vi "The ChapR.vi"(8 "Digtl In":u8, 9 "Position":u8=49, 10 "Alliance":u8=66, 11 "TeamNo":u16) -> ()   [LabVIEW 2013]
uses:
  ChapR Packet.ctl
  <vilib>/Instr/_visa.llb/VISA Configure Serial Port (Instr).vi
panel:
  out "error out 3":errorcluster
  in  "connection ID":refnum<k16>
  out "error out 2":errorcluster
  out "# elements 2":u32
  out "# elements":u32
  out "error out":errorcluster
  out "value 2":T1
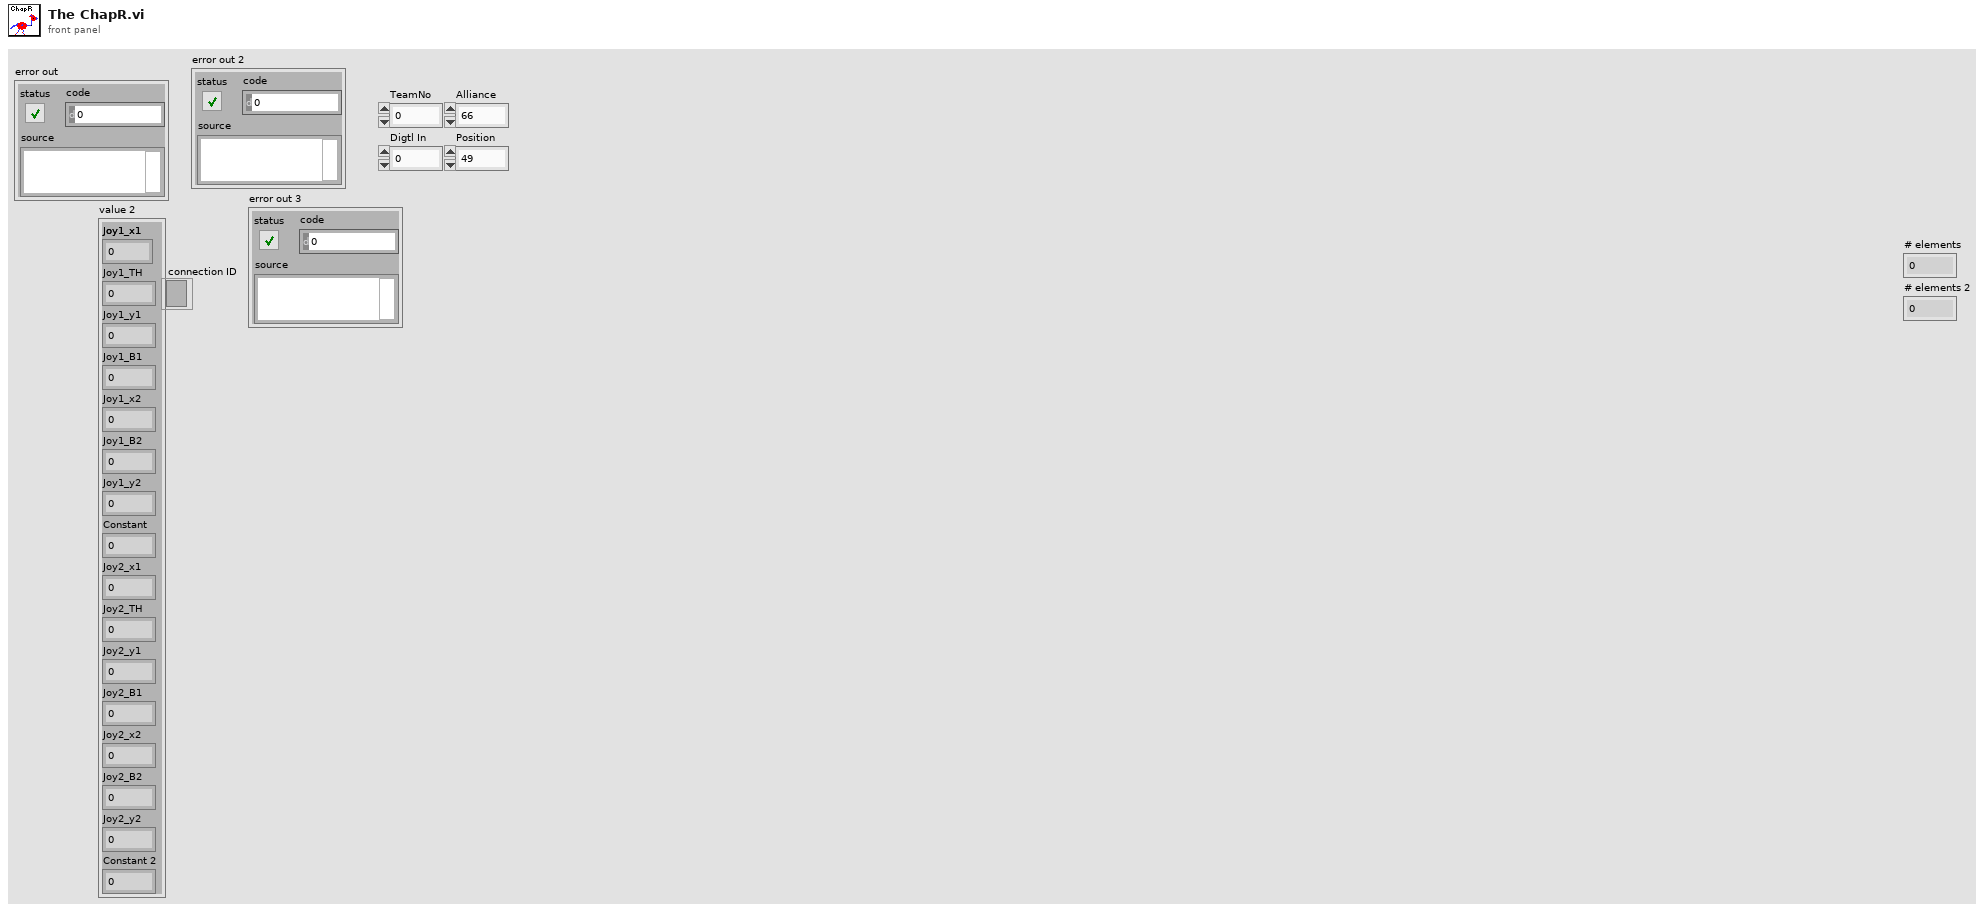
[diagram p1: front panel]
types:
  T1 = typedef "ChapR Packet.ctl" = cluster{"Joy1_x1":i8, "Joy1_TH":u8, "Joy1_y1":i8, "Joy1_B1":u8, "Joy1_x2":i8, "Joy1_B2":u8, "Joy1_y2":i8, "Constant":u8, "Joy2_x1":i8, "Joy2_TH":u8, "Joy2_y1":i8, "Joy2_B1":u8, "Joy2_x2":i8, "Joy2_B2":u8, "Joy2_y2":i8, "Constant 2":u8}
  T2 = cluster{"read mode":enum16{"polling", "blocking"}, "write mode":enum16{"polling", "blocking"}}
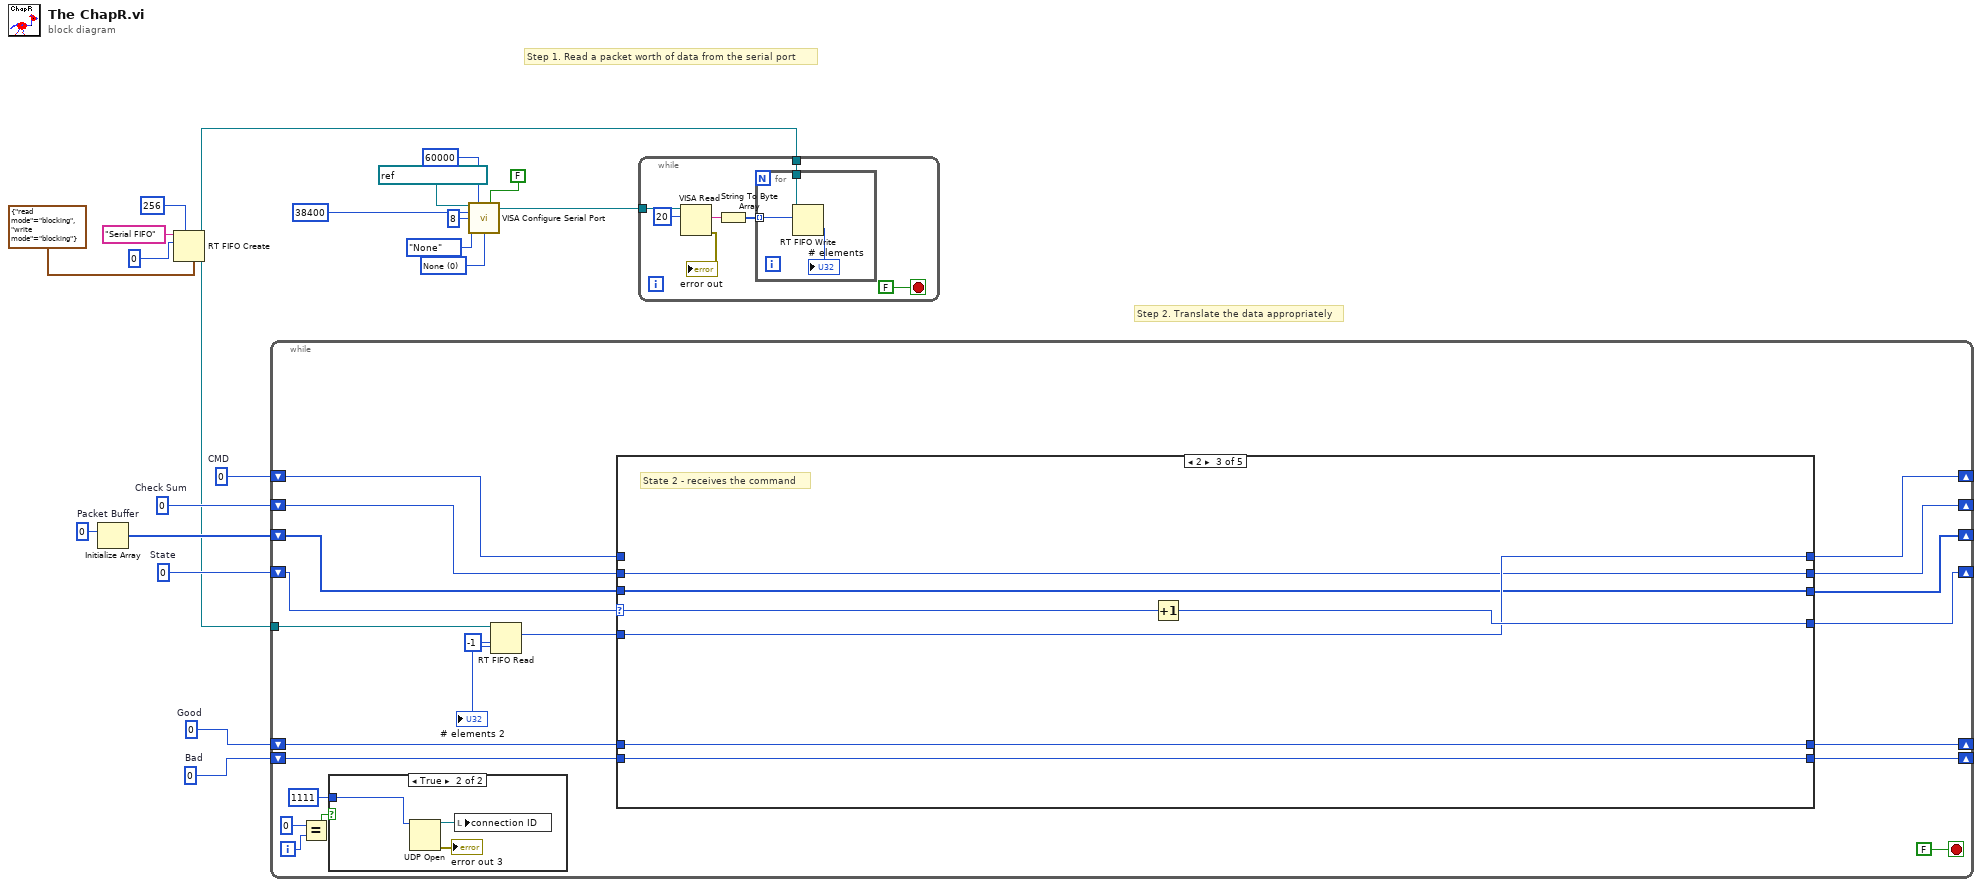
[diagram p0: block diagram]
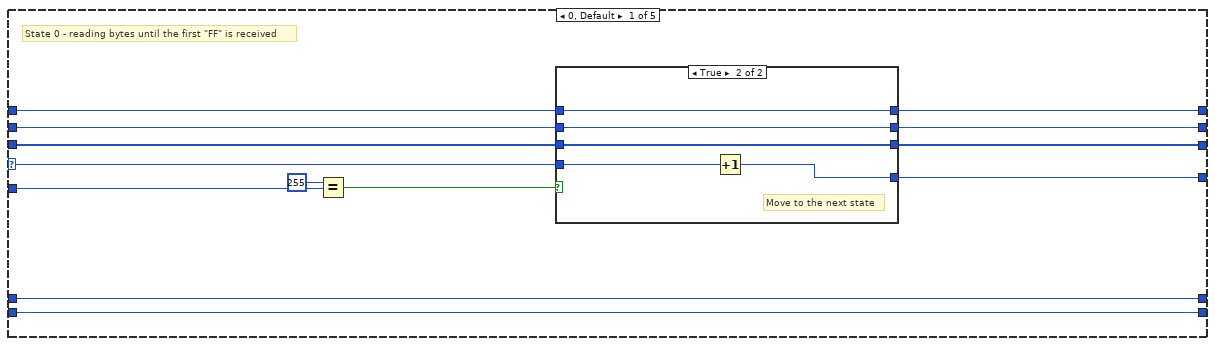
[diagram p3: hidden frame]
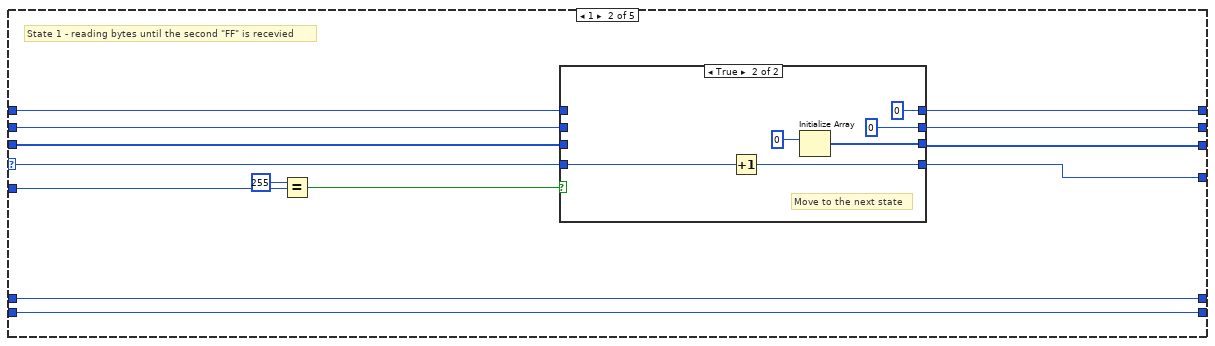
[diagram p5: hidden frame]
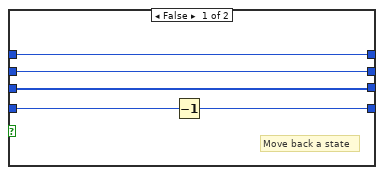
[diagram p6: hidden frame]
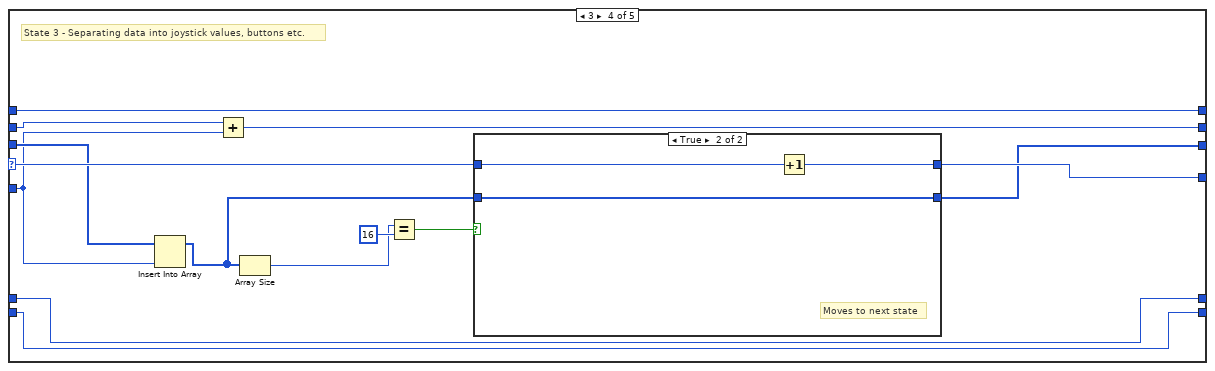
[diagram p7: hidden frame]
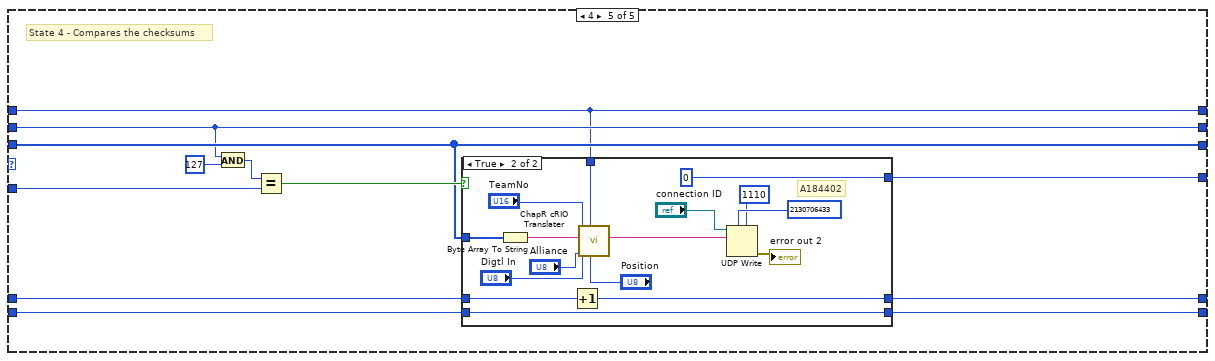
[diagram p9: hidden frame]
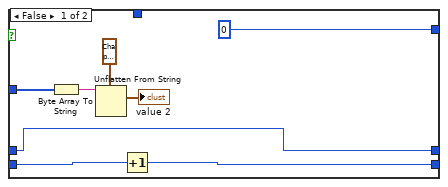
[diagram p10: hidden frame]
diagram:
  w5 = 0  # Bad
  w6 = 0  # Good
  w19 = u16 0 items=["None", "XON/XOFF", "RTS/CTS", "XON/XOFF & RTS/CTS", "DTR/DSR", "XON/XOFF & DTR/DSR"] ("flow control (0:none)")
  w3 = u8 0  # CMD
  w4 = u8 0  # Check Sum
  w20 = 0  # State
  # "Step 2. Translate the data appropriately"
  # "Step 1. Read a packet worth of data from the serial port"
  n1 = Initialize Array "Packet Buffer"(u8 0 ("element")) -> (w8:u8[])  [unwired: 1 in]
  n2 = RT FIFO Create(0:"Serial FIFO" ("name (unnamed)"), 1:u8 0 ("datapoints in waveform (1)"), 4:u32 256 ("size (10)"), 7:T2 {"read mode"=enum."blocking", "write mode"=enum."blocking"} ("r/w modes (polling,polling)")) -> (8:w1:refnum<k33>)  [unwired: 4 in, 2 out]
  n3 = while {
    shift-right: [w39] -> _
    shift-left: w20 -> [w40]
    shift-right: [w29] -> _
    shift-left: w4 -> [w30]
    tunnel: w1 -> [w37]
    shift-right: [w35] -> _
    shift-left: w8 -> [w36]
    shift-right: [w31] -> _
    shift-left: w6 -> [w34]
    shift-right: [w32] -> _
    shift-left: w5 -> [w33]
    shift-right: [w27] -> _
    shift-left: w3 -> [w28]
    i -> [w23]
    stop <- FALSE stop-if-true
    n4 = Equal?(x=0, y=w23) -> (x = y?=w24:bool)
    n5 = case shown="True" w24 {
      tunnel: u16 1111 ("port") -> [_ w43]
      frame False {
      }
      frame True {
        n6 = UDP Open(11:w43) -> (port=w44:refnum<k16>, 0:→"error out 3":errorcluster)  [unwired: 4 in, 1 out]
        n7 = local write "connection ID"(w44) -> ()
      }
    }
    n8 = RT FIFO Read(0:w37, 2:-1 ("timeout in ms (0)")) -> (7:→"# elements 2":u32, 9:w38:u8)  [unwired: 2 in, 3 out]
    n9 = case shown="2" w40 {
      selector: w40 -> [w56 w79 w97 w110 _]
      tunnel: [w55 w78 w96 w111 w127] -> w39
      tunnel: [w47 w69 w91 w108 w118] -> w29
      tunnel: [w45 w67 w95 w98 w117] -> w27
      tunnel: w38 -> [w53 w75 w95 w106 w124]
      tunnel: w36 -> [w52 w73 w94 w107 w123]
      tunnel: [w51 w74 w94 w102 w123] -> w35
      tunnel: w34 -> [w50 w72 w93 w101 w120]
      tunnel: w33 -> [w49 w71 w92 w100 w122]
      tunnel: [w49 w71 w92 w100 w121] -> w32
      tunnel: [w50 w72 w93 w101 w119] -> w31
      tunnel: w30 -> [w48 w70 w91 w99 w118]
      tunnel: w28 -> [w46 w68 _ w98 w117]
      frame 0, Default {
        # "State 0 - reading bytes until the first \"FF\" is received"
        n10 = Equal?(x=u8 255, y=w53) -> (x = y?=w57:bool)
        n11 = case shown="True" w57 {
          tunnel: w56 -> [w61 w66]
          tunnel: [w61 w65] -> w55
          tunnel: w52 -> [w60 w64]
          tunnel: [w60 w64] -> w51
          tunnel: [w59 w63] -> w47
          tunnel: w48 -> [w59 w63]
          tunnel: [w58 w62] -> w45
          tunnel: w46 -> [w58 w62]
          frame False {
            # "Do nothing"
          }
          frame True {
            # "Move to the next state"
            n12 = Increment(x=w66) -> (x+1=w65:i32)
          }
        }
      }
      frame 1 {
        # "State 1 - reading bytes until the second \"FF\" is recevied"
        n13 = Equal?(x=u8 255, y=w75) -> (x = y?=w76:bool)
        n14 = case shown="True" w76 {
          tunnel: [w83 w89] -> w78
          tunnel: w79 -> [w84 w90]
          tunnel: [w81 u8 0] -> w69
          tunnel: [w80 u8 0] -> w67
          tunnel: [w82 w85] -> w74
          tunnel: w73 -> [w82 _]
          tunnel: w70 -> [w81 _]
          tunnel: w68 -> [w80 _]
          frame False {
            # "Move back a state"
            n15 = Decrement(x=w84) -> (x-1=w83:i32)
          }
          frame True {
            # "Move to the next state"
            n16 = Increment(x=w90) -> (x+1=w89:i32)
            n17 = Initialize Array ("Packet Buffer")(u8 0 ("element")) -> (w85:u8[])  [unwired: 1 in]
          }
        }
      }
      frame 2 {
        # "State 2 - receives the command"
        n18 = Increment(x=w97) -> (x+1=w96:i32)
      }
      frame 3 {
        # "State 3 - Separating data into joystick values, buttons etc."
        n19 = Insert Into Array(array=w107, new element=w106) -> (w103:u8[])  [unwired: 1 in]
        n20 = Add(x=w99, y=w106) -> (x+y=w108:u8)
        n21 = Array Size(array=w103) -> (size(s)=w105:i32)
        n22 = Equal?(x=w105, y=16) -> (x = y?=w104:bool)
        n23 = case shown="True" w104 {
          tunnel: [w113 w115] -> w111
          tunnel: w110 -> [w113 w116]
          tunnel: w103 -> [w112 w114]
          tunnel: [w112 w114] -> w102
          frame False {
            # "Do nothing"
          }
          frame True {
            # "Moves to next state"
            n24 = Increment(x=w116) -> (x+1=w115:i32)
          }
        }
      }
      frame 4 {
        # "State 4 - Compares the checksums"
        n25 = And(x=w118, y=u8 127) -> (x .and. y?=w126:u8)
        n26 = Equal?(x=w126, y=w124) -> (x = y?=w128:bool)
        n27 = case shown="True" w128 {
          tunnel: [0 0] -> w127
          tunnel: w123 -> [w134 w151]
          tunnel: w122 -> [w132 w150]
          tunnel: [w131 w150] -> w121
          tunnel: w120 -> [w130 w149]
          tunnel: [w130 w148] -> w119
          tunnel: w117 -> [_ w137]
          frame False {
            n28 = Byte Array To String(unsigned byte array=w134) -> (string=w133:string)
            n29 = Unflatten From String(type=T1 {"Joy1_x1"=0, "Joy1_TH"=0, "Joy1_y1"=0, "Joy1_B1"=0, "Joy1_x2"=0, "Joy1_B2"=0, "Joy1_y2"=0, "Constant"=0, "Joy2_x1"=0, "Joy2_TH"=0, "Joy2_y1"=0, "Joy2_B1"=0, "Joy2_x2"=0, "Joy2_B2"=0, "Joy2_y2"=0, "Constant 2"=0}, binary string=w133) -> (value=→"value 2":T1)  [unwired: 3 in, 2 out]
            n30 = Increment(x=w132) -> (x+1=w131:i32)
          }
          frame True {
            # "A184402"
            n31 = Byte Array To String(unsigned byte array=w151) -> (string=w147:string)
            n32 = Increment(x=w149) -> (x+1=w148:i32)
            n33 = call "ChapR cRIO Translater.vi"("Position"="Position", "CMD"=w137, "Alliance"="Alliance", "Digtl In"="Digtl In", "ChapR Data"=w147, "TeamNo"="TeamNo") -> ("Network Data"=w140:string)  [unwired: 5 in]
            n34 = UDP Write(address=u32 2130706433 ("net address"), port or service name=u16 1110, connection ID="connection ID", data in=w140) -> (error out=→"error out 2":errorcluster)  [unwired: 2 in, 1 out]
          }
        }
      }
    }
  }
  n35 = call-poly "VISA Configure Serial Port"("VISA resource name"=refnum<visa-resource-name> "ASRL1::INSTR", "timeout (10sec)"=u32 60000, "Enable Termination\nChar (T)"=FALSE ("Enable Termination\nChar (T)"), "baud rate (9600)"=u32 38400, "data bits (8)"=u16 8, "parity (0:none)"=enum16{"None", "Odd", "Even", "Mark", "Space"}."None", "flow control (0:none)"=w19) -> ("VISA resource name out"=w12:refnum<visa-resource-name>)  [unwired: 7 in, 1 out]
  n36 = while {
    tunnel: w12 -> [w158]
    tunnel: w1 -> [w156]
    stop <- FALSE stop-if-true
    n37 = VISA Read(VISA resource name=w158, byte count=u32 20) -> (read buffer=w154:string, error out=→"error out":errorcluster)  [unwired: 1 in, 2 out]
    n38 = String To Byte Array(string=w154) -> (unsigned byte array=w155:u8[])
    n39 = for {
      tunnel: w156 -> [w162]
      tunnel: w155 -> [w161] mode=indexing
      n40 = RT FIFO Write(0:w162, 1:w161) -> (7:→"# elements":u32)  [unwired: 3 in, 3 out]
    }
  }
